vi "Start Run.vi"(6 "clone#":i32, 8 "done ref":refnum<vi>, 11 "NetCPU in":refnum<class "NetCPU.lvclass">) -> (3 "NetCPU out":refnum<class "NetCPU.lvclass">)   [LabVIEW 2020, in "NI_TargetHelper.lvlib" / "NetCPU.lvclass"]
uses:
  <vilib>/TargetSupport/NI_TargetHelper/NetCPU/NetCPU.lvclass
  <vilib>/TargetSupport/NI_TargetHelper/NetCPU/NetCPU.lvclass/NetCPU.ctl
  <vilib>/TargetSupport/NI_TargetHelper/Run Target VI.ctl
  <vilib>/TargetSupport/NI_TargetHelper/NI_TargetHelper.lvlib
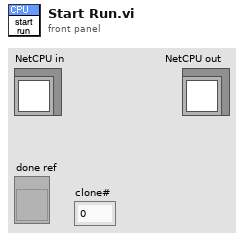
[diagram p1: front panel]
types:
  T1 = typedef "NI_TargetHelper.lvlib/Run Target VI.ctl" = refnum<vi>
  T2 = typedef "NI_TargetHelper.lvlib/Instance VIref.ctl" = refnum<vi>
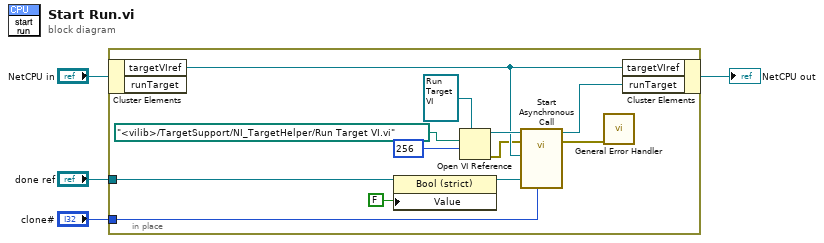
[diagram p0: block diagram]
diagram:
  n1 = in-place {
    in-place-border: "done ref" -> [w9]
    in-place-border: "clone#" -> [w8]
    n2 = in-place-cluster #1("NetCPU in") -> ("targetVIref"=w10:T2)  [unwired: 1 out]
    n3 = property class="Bool (strict)"(reference=w9, "Value"=FALSE) -> (reference out=w12:refnum<vi>)  [unwired: 1 in, 1 out]
    n4 = Open VI Reference(type specifier VI Refnum (for type only)=T1 refnum ("runTarget"), vi path=path "<vilib>/TargetSupport/NI_TargetHelper/Run Target VI.vi", options=256) -> (vi reference=w14:T1, error out=w6:errorcluster)  [unwired: 3 in]
    n5 = call-by-ref "Start Asynchronous Call"(reference=w14, error in=w6, "clone#"=w8, "doneRef"=w12, "targetVIref"=w10) -> (reference out=w11:T1, error out=w5:errorcluster)  [unwired: 9 in]
    n6 = call <vilib>:"General Error Handler.vi"("error in (no error)"=w5) -> ()  [unwired: 10 in, 5 out]
    n7 = in-place-cluster #1("targetVIref"=w10, "runTarget"=w11) -> (→"NetCPU out":refnum<class "NetCPU.lvclass">)
  }
